vi "MH_Graph_DeltasClass.vi"() -> ()   [LabVIEW 2019]
uses:
  <userlib>/MultiHarp150/T2Lib/MH_T2DeltaQMessage.ctl
panel:
  out "Deltas":i32[](array[numeric])
  out "delta processed":i32
  in  "stop":bool
  in  "WindowWidth":u32
  out "Correlations":u32[](array[numeric])
  in  "BinSize":u32
  in  "ErrorIn":errorcluster caption="entrée d'erreur (pas d'erreur)"
  out "Graph":u32[](graph)
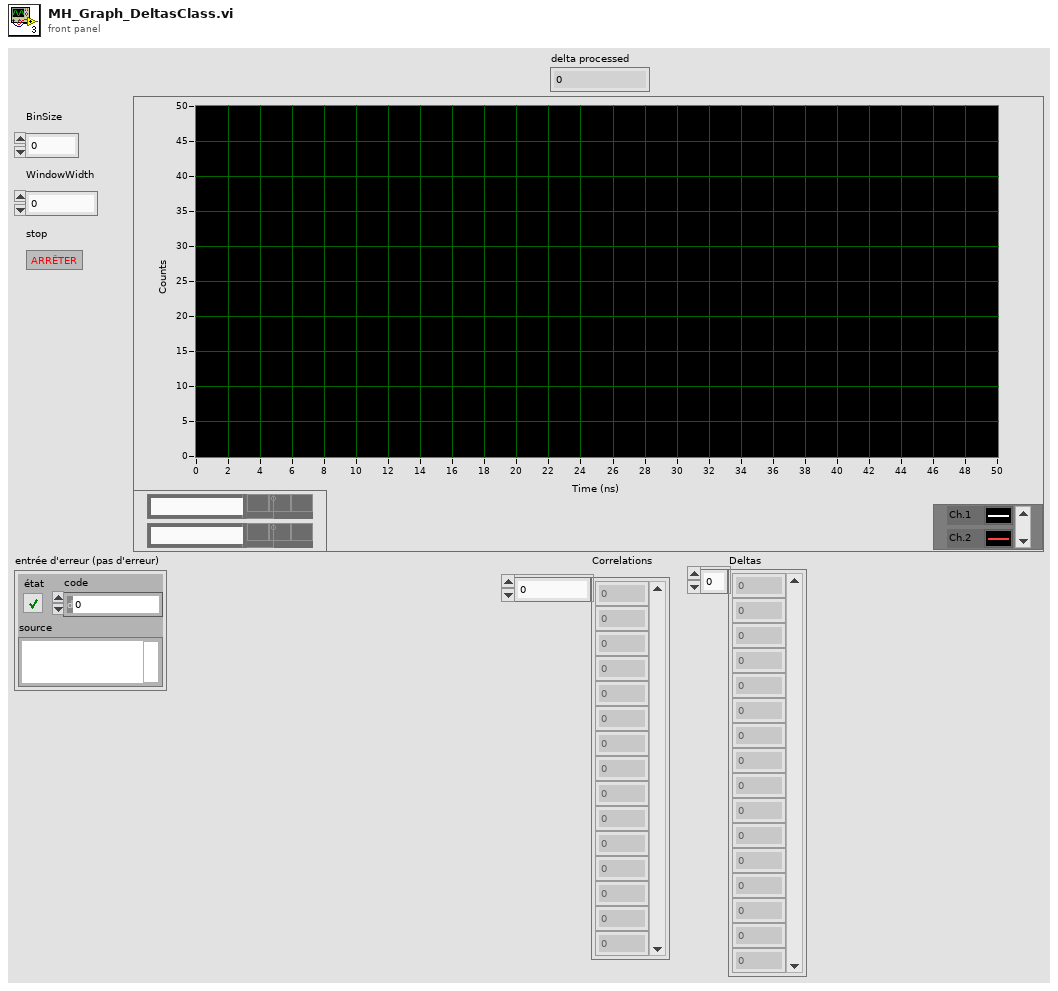
[diagram p1: front panel]
types:
  T1 = typedef "MH_T2DeltaQMessage.ctl" = cluster{"Message":string, "buffer":i32[], "Code":i32, "nactual":i32}
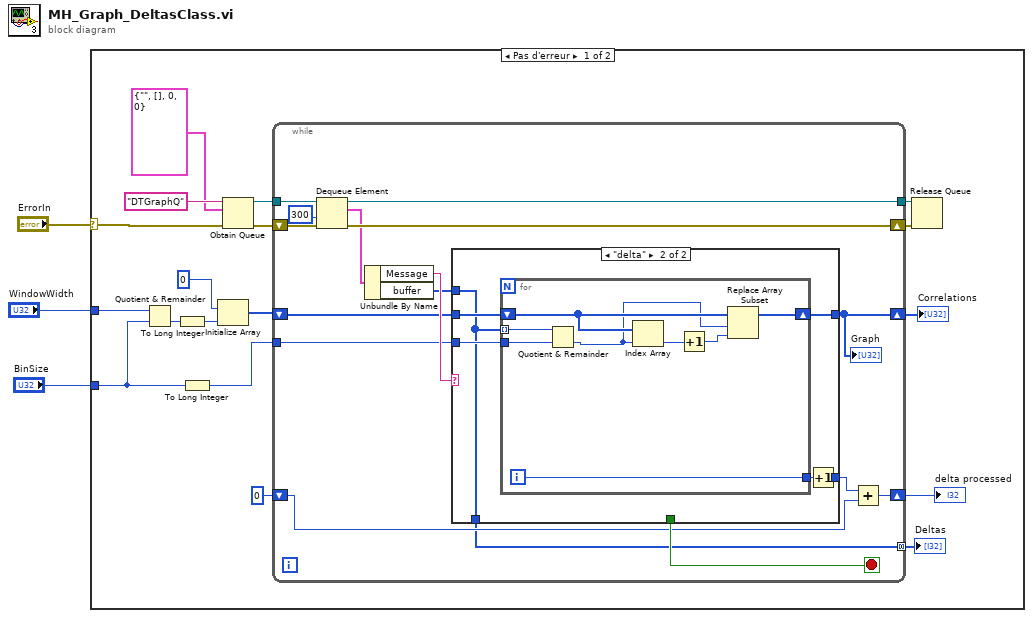
[diagram p0: block diagram]
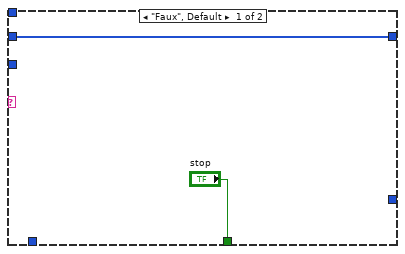
[diagram p2: hidden frame]
diagram:
  n1 = case shown="Pas d'erreur" "ErrorIn" {
    selector: "ErrorIn" -> [w15 _]
    tunnel: "BinSize" -> [w12 _]
    tunnel: "WindowWidth" -> [w13 _]
    frame No Error {
      n2 = Quotient & Remainder(x=w13, y=w12) -> (floor(x/y)=w11:u32)  [unwired: 1 out]
      n3 = To Long Integer(number=w11) -> (32bit integer=w10:i32)
      n4 = To Long Integer(number=w12) -> (32bit integer=w4:i32)
      n5 = Initialize Array(u32 0 ("WindowWidth"), w10) -> (w8:u32[])
      n6 = Obtain Queue(name (unnamed)="DTGraphQ" ("nom (aucun)"), element data type=T1 {"Message"="", "buffer"=[], "Code"=0, "nactual"=0} ("ClassQueue"), error in (no error)=w15) -> (queue out=w18:refnum<queue>, error out=w19:errorcluster)  [unwired: 2 in, 1 out]
      n7 = while {
        tunnel: w18 -> [w36]
        shift-right: [w35] -> w17
        shift-left: w19 -> [w37]
        tunnel: [w34] -> w16
        tunnel: w4 -> [w31]
        shift-right: [w28] -> w14
        shift-left: w8 -> [w30]
        shift-right: [w24] -> w5
        shift-left: 0 -> [w23]
        tunnel: [w22] -> w6 mode=concatenating
        stop <- w27 stop-if-true
        n8 = Dequeue Element(queue=w36, timeout in ms (-1)=300 ("timeout en ms (-1)"), error in (no error)=w37) -> (queue out=w34:refnum<queue>, element=w33:T1, error out=w35:errorcluster)  [unwired: 1 out]
        n9 = Unbundle By Name(w33) -> ("Message"=w32:string, "buffer"=w29:i32[])
        n10 = case shown="\"delta\"" w32 {
          tunnel: w31 -> [_ w45]
          tunnel: w30 -> [w39 w44]
          tunnel: [w39 w43] -> w28
          tunnel: w29 -> [_ w41]
          tunnel: ["stop" _] -> w27
          tunnel: [_ w40] -> w25
          tunnel: [_ w41] -> w22
          frame "Faux", Default {
          }
          frame "delta" {
            n11 = for {
              tunnel: w41 -> [w47] mode=indexing
              tunnel: w45 -> [w53]
              shift-right: [w49] -> w43
              shift-left: w44 -> [w50]
              tunnel: [w48] -> w42
              i -> [w48]
              n12 = Quotient & Remainder(x=w47, y=w53) -> (floor(x/y)=w46:i32)  [unwired: 1 out]
              n13 = Index Array(array=w50, index=w46) -> (element=w52:u32)
              n14 = Increment(x=w52) -> (x+1=w51:u32)
              n15 = Replace Array Subset(array=w50, new element=w51, index=w46) -> (w49:u32[])
            }
            n16 = Increment(x=w42) -> (x+1=w40:i32)
          }
        }
        "Graph" <- w28
        n17 = Add(x=w25, y=w23) -> (x+y=w24:i32)
      }
      "Correlations" <- w14
      "delta processed" <- w5
      "Deltas" <- w6
      n18 = Release Queue(queue=w16, error in (no error)=w17) -> ()  [unwired: 1 in, 3 out]
    }
    frame Error {
    }
  }
